vi "ODMR sweep new locked.vi"() -> ()   [LabVIEW 2011]
uses:
  <vilib>/DAQmx/read.llb/DAQmx Read (Counter 1D DBL 1Chan NSamp).vi
  <vilib>/DAQmx/write.llb/DAQmx Write (Digital Bool 1Line 1Point).vi
  <vilib>/DAQmx/create/channels.llb/DAQmx Create Channel (DO-Digital Output).vi
  <vilib>/DAQmx/create/channels.llb/DAQmx Create Channel (CI-Count Edges).vi
  <vilib>/DAQmx/configure/timing.llb/DAQmx Timing (Sample Clock).vi
  <vilib>/Utility/file.llb/Write To Spreadsheet File (DBL).vi
  <vilib>/DAQmx/miscellaneous.llb/DAQmx Fill In Error Info.vi
  Program Files/National Instruments/LabVIEW 2011/resource/objmgr/daqmx.rc
panel:
  out "Frequency":dbl
  in  "Freq max":ext=3300000000.0
  in  "Tracking interval":dbl=150.0
  out "XY Graph":cluster{"Y":dbl[], "Y":dbl[]}[](graph)
  in  "band (1-26.5:2) 2":i32(ring)=2
  in  "resolution (10 Hz:2) 2":i32(ring)=2 items=["0.1 Hz", "1 Hz", "10 Hz", "100 Hz", "1 KHz", "10 KHz", "100 KHz", "1 MHz", "10 MHz", "100 MHz", "1 GHz"]
  in  "GPIB address 2":string="19"
  in  "file path (dialog if empty)":path=path "C:/Users/Ouyang Group/Documents/Calibration pictures/Nanodiamond/1-8-14/X=66 Y=92 Pulse ODMR sweep 4"
  out "Z Position":dbl=31.0
  out "Y Position":dbl=62.0
  out "X Position":dbl=97.0
  in  "Z Pos":dbl=31.0
  in  "Y Pos":dbl=97.0
  in  "X Pos":dbl=62.0
  in  "Y Parameters":T1={"Number of Y Steps"=200, "Max Y (V)"=1.0, "Min Y (V)"=-1.0}
  in  "X Parameters":T2={"Number of X Steps"=200, "Max X (V)"=1.0, "Min X (V)"=-1.0}
  in  "RS232 settings":cluster{"Portnumber":i32, "Baudrate":u16}={"Portnumber"=12, "Baudrate"=5} {"Portnumber" items=["COM1", "COM2", "COM3", "COM4", "COM5", "COM6", "COM7", "COM8", "COM9", "COM10", "COM11", "COM12", "COM13", "COM14", "COM15", "COM16", "COM17", "COM18", "COM19", "COM20", "COM21", "COM22", "COM23", "COM24", "COM25", "COM26", "COM27", "COM28", "COM29", "COM30"]; "Baudrate" items=["9600", "14400", "19200", "38400", "57600", "115200"]}
  in  "samples per channel":i32=500
  in  "rate":dbl=100.0 format="%0.2f"
  in  "stop":bool
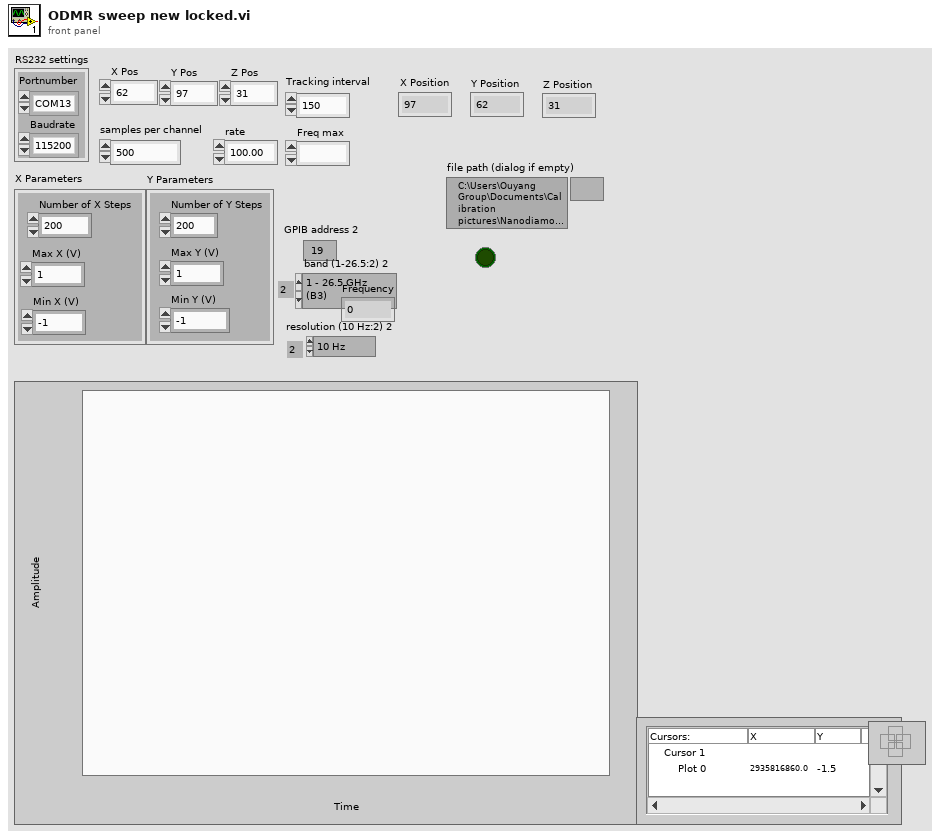
[diagram p1: front panel]
types:
  T1 = cluster{"Number of Y Steps":i32, "Max Y (V)":dbl, "Min Y (V)":dbl}
  T2 = cluster{"Number of X Steps":i32, "Max X (V)":dbl, "Min X (V)":dbl}
  T3 = cluster{"source lock":bool, "lock frequency (Hz)":ext, "coarse tune":bool}
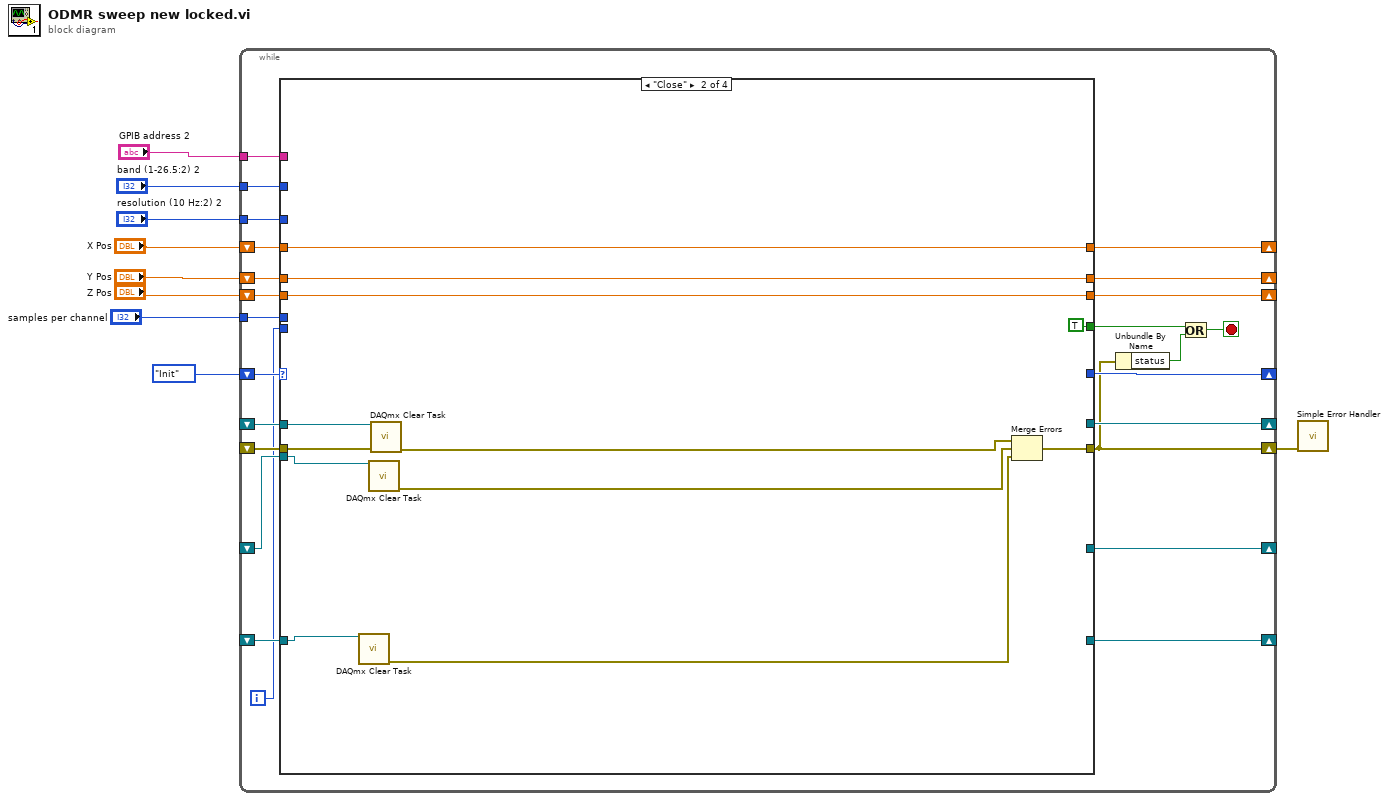
[diagram p0: block diagram]
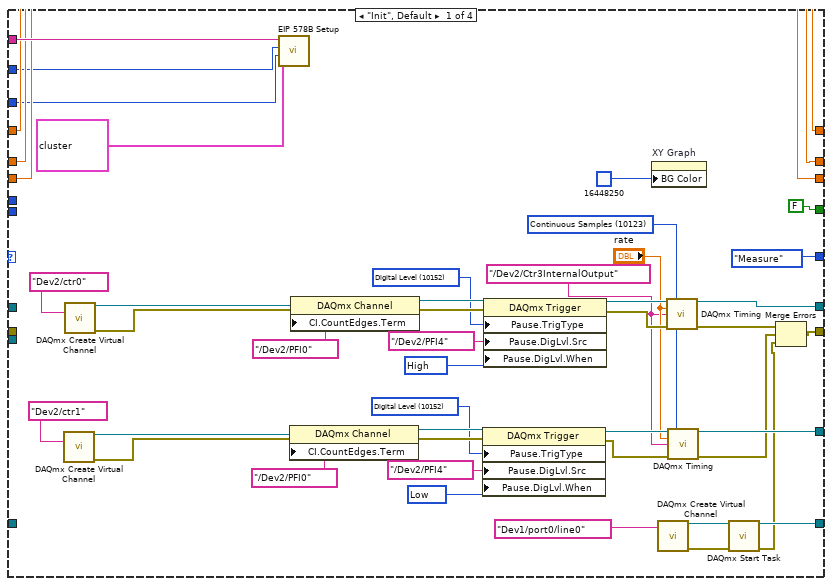
[diagram p2: hidden frame]
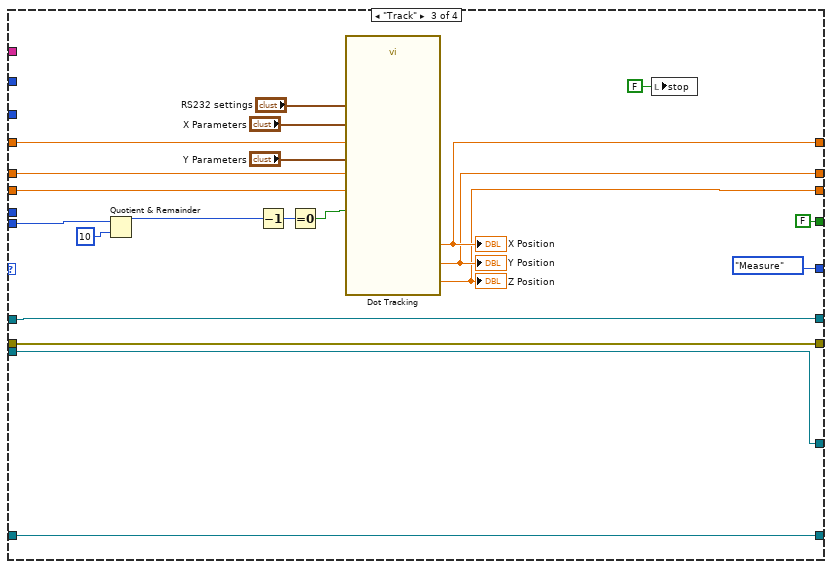
[diagram p3: hidden frame]
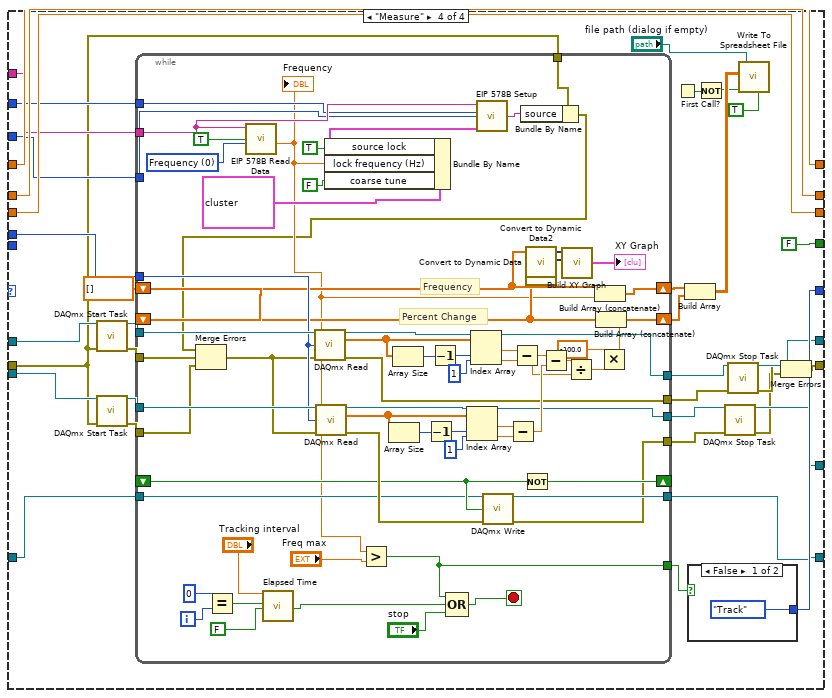
[diagram p4: hidden frame]
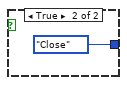
[diagram p5: hidden frame]
diagram:
  n1 = while {
    shift-right: [w29] -> _
    shift-left: enum16{"Init", "Measure", "Track", "Close"}."Init" -> [w33]
    tunnel: "GPIB address 2" -> [w32]
    shift-right: [w31] -> _
    shift-left: _ -> [w28]
    shift-right: [w30] -> _
    shift-left: _ -> [w27]
    shift-right: [w22] -> w6
    shift-left: _ -> [w26]
    shift-right: [w25] -> _
    shift-left: _ -> [w24]
    tunnel: "samples per channel" -> [w19]
    shift-right: [w14] -> _
    shift-left: "X Pos" -> [w17]
    shift-right: [w13] -> _
    shift-left: "Y Pos" -> [w16]
    shift-right: [w12] -> _
    shift-left: "Z Pos" -> [w15]
    tunnel: "band (1-26.5:2) 2" -> [w11]
    tunnel: "resolution (10 Hz:2) 2" -> [w10]
    i -> [w23]
    stop <- w21 stop-if-true
    n2 = case shown="\"Close\"" w33 {
      tunnel: [FALSE TRUE FALSE FALSE] -> w20
      tunnel: w32 -> [w77 _ _ w116]
      tunnel: [w51 _ w111 w134] -> w31
      tunnel: [w50 _ w110 w131] -> w30
      tunnel: [w47 w83 w100 w147] -> w22
      tunnel: [enum16{"Init", "Measure", "Track", "Close"}."Measure" _ enum16{"Init", "Measure", "Track", "Close"}."Measure" w146] -> w29
      tunnel: w28 -> [_ w89 w111 w142]
      tunnel: w27 -> [_ w87 w110 w139]
      tunnel: w26 -> [_ w88 w100 w113]
      tunnel: [w41 _ w109 w135] -> w25
      tunnel: w24 -> [_ w86 w109 w136]
      tunnel: w23 -> [_ _ w101 _]
      tunnel: w19 -> [_ _ _ w121]
      tunnel: w17 -> [w38 w81 w96 w119]
      tunnel: w16 -> [w37 w80 w95 w118]
      tunnel: w15 -> [w36 w79 w94 w117]
      tunnel: [w38 w81 w93 w119] -> w14
      tunnel: [w37 w80 w92 w118] -> w13
      tunnel: [w36 w79 w91 w117] -> w12
      tunnel: w11 -> [w35 _ _ w115]
      tunnel: w10 -> [w34 _ _ w114]
      frame "Init", Default {
        w52 = tag "/Dev2/Ctr3InternalOutput" ("source")
        w54 = 10123 items=["Finite Samples"=10178, "Continuous Samples"=10123, "Hardware Timed Single Point"=12522] ("sample mode")
        w59 = 10214 items=["High"=10192, "Low"=10214] ("Pause.DigLvl.When")
        w61 = 10152 items=["Analog Level"=10101, "Analog Window"=10103, "Digital Level"=10152, "Digital Pattern"=10398, "None"=10230] ("Pause.TrigType")
        w68 = 10192 items=["High"=10192, "Low"=10214] ("Pause.DigLvl.When")
        w70 = 10152 items=["Analog Level"=10101, "Analog Window"=10103, "Digital Level"=10152, "Digital Pattern"=10398, "None"=10230] ("Pause.TrigType")
        n3 = call-poly <vilib>:"DAQmx Create Virtual Channel.vi"("counter"=tag "Dev2/ctr1") -> ("task out"=w66:refnum<k21>, "error out"=w65:errorcluster)  [unwired: 13 in]
        n4 = call-poly <vilib>:"DAQmx Create Virtual Channel.vi"("counter"=tag "Dev2/ctr0") -> ("task out"=w75:refnum<k21>, "error out"=w74:errorcluster)  [unwired: 13 in]
        n5 = call <instrlib>:"EIP 578B Setup.vi"("GPIB Address"=w77, "band (1-26.5 GHz:20)"=w35, "resolution (1 Hz:1)"=w34, "source locking"=T3 {"source lock"=FALSE, "lock frequency (Hz)"=1000000000.0, "coarse tune"=TRUE}) -> ()  [unwired: 2 in, 2 out]
        n6 = property class="DAQmx Channel"(reference=w66, error in=w65, "CI.CountEdges.Term"=tag "/Dev2/PFI0") -> (reference out=w63:refnum<k21>, error out=w62:errorcluster)
        n7 = property class="DAQmx Channel"(reference=w75, error in=w74, "CI.CountEdges.Term"=tag "/Dev2/PFI0") -> (reference out=w72:refnum<k21>, error out=w71:errorcluster)
        n8 = property class="DAQmx Trigger"(reference=w63, error in=w62, "Pause.TrigType"=w61, "Pause.DigLvl.Src"=tag "/Dev2/PFI4", "Pause.DigLvl.When"=w59) -> (reference out=w56:refnum<k21>, error out=w55:errorcluster)
        n9 = property class="DAQmx Trigger"(reference=w72, error in=w71, "Pause.TrigType"=w70, "Pause.DigLvl.Src"=tag "/Dev2/PFI4", "Pause.DigLvl.When"=w68) -> (reference out=w58:refnum<k21>, error out=w57:errorcluster)
        n10 = property on="XY Graph" class="XYGraph (strict)"("BG Color"=u32 16448250) -> ()  [unwired: 2 in, 2 out]
        n11 = call-poly <vilib>:"DAQmx Create Virtual Channel.vi"("lines"=tag "Dev1/port0/line0") -> ("task out"=w43:refnum<k21>, "error out"=w42:errorcluster)  [unwired: 13 in]
        n12 = call-poly <vilib>:"DAQmx Timing.vi"("task/channels in"=w58, "sample mode"=w54, "rate"="rate", "source"=w52, "error in"=w57) -> ("task out"=w51:refnum<k21>, "error out"=w49:errorcluster)  [unwired: 9 in]
        n13 = call-poly <vilib>:"DAQmx Timing.vi"("task/channels in"=w56, "sample mode"=w54, "rate"="rate", "source"=w52, "error in"=w55) -> ("task out"=w50:refnum<k21>, "error out"=w48:errorcluster)  [unwired: 9 in]
        n14 = call <vilib>:"DAQmx Start Task.vi"("task/channels in"=w43, "error in"=w42) -> ("task out"=w41:refnum<k21>, "error out"=w40:errorcluster)  [unwired: 12 in]
        n15 = Merge Errors(w49, w48, w40) -> (w47:errorcluster)
      }
      frame "Close" {
        n16 = call <vilib>:"DAQmx Clear Task.vi"("task in"=w86) -> ("error out"=w84:errorcluster)  [unwired: 14 in]
        n17 = call <vilib>:"DAQmx Clear Task.vi"("task in"=w87) -> ("error out"=w85:errorcluster)  [unwired: 14 in]
        n18 = call <vilib>:"DAQmx Clear Task.vi"("task in"=w89, "error in"=w88) -> ("error out"=w82:errorcluster)  [unwired: 13 in]
        n19 = Merge Errors(w82, w85, w84) -> (w83:errorcluster)
      }
      frame "Track" {
        n20 = Quotient & Remainder(x=w101, y=10) -> (x-y*floor(x/y)=w104:i32)  [unwired: 1 out]
        n21 = Decrement(x=w104) -> (x-1=w105:i32)
        n22 = Equal To 0?(x=w105) -> (x = 0?=w102:bool)
        n23 = call "Dot Tracking.vi"("X Parameters"="X Parameters", "Y Parameters"="Y Parameters", "RS232 settings"="RS232 settings", "X Pos"=w96, "Y pos"=w95, "Z Pos"=w94, "Z-track?"=w102) -> ("X Position"=w93:dbl, "Y Position"=w92:dbl, "Z Position"=w91:dbl)  [unwired: 2 in, 4 out]
        "X Position" <- w93
        "Y Position" <- w92
        "Z Position" <- w91
        n24 = local write "stop"(FALSE ("stop")) -> ()
      }
      frame "Measure" {
        w120 = dbl[] []
        n25 = call <vilib>:"DAQmx Start Task.vi"("task/channels in"=w142, "error in"=w113) -> ("task out"=w140:refnum<k21>, "error out"=w141:errorcluster)  [unwired: 12 in]
        n26 = call <vilib>:"DAQmx Start Task.vi"("task/channels in"=w139, "error in"=w113) -> ("task out"=w138:refnum<k21>, "error out"=w137:errorcluster)  [unwired: 12 in]
        n27 = while {
          shift-right: [w199] -> w127
          shift-left: w120 -> [w179]
          shift-right: [w198] -> w128
          shift-left: w120 -> [w181]
          shift-right: [w192] -> _
          shift-left: _ -> [w193]
          tunnel: w138 -> [w191]
          tunnel: [w190] -> w133
          tunnel: [w189] -> w144
          tunnel: [w184] -> w143
          tunnel: w141 -> [w188]
          tunnel: w140 -> [w187]
          tunnel: w137 -> [w152]
          tunnel: w136 -> [w186]
          tunnel: [w185] -> w135
          tunnel: [w183] -> w130
          tunnel: w121 -> [w182]
          tunnel: w116 -> [w166]
          tunnel: w115 -> [w165]
          tunnel: w114 -> [w164]
          tunnel: w113 -> [w155]
          tunnel: [w150] -> w112
          i -> [w168]
          stop <- w156 stop-if-true
          w172 = 0 items=["Frequency", "Power", "Both"] ("output mode (freq:0)")
          # "Percent Change"
          # "Frequency"
          n28 = Equal?(x=0, y=w168) -> (x = y?=w167:bool)
          n29 = call <instrlib>:"EIP 578B Read Data.vi"("output mode (freq:0)"=w172, "fast (T=active)"=TRUE, "GPIB"=w166) -> ("frequency (Hz)"=w159:ext)  [unwired: 1 in, 3 out]
          "Frequency" <- w159
          n30 = call "Elapsed Time"("Time Target (s)"="Tracking interval", "Reset"=w167, "Auto Reset"=FALSE) -> ("Time has Elapsed"=w158:bool)  [unwired: 9 in, 7 out]
          n31 = Bundle By Name(cluster=T3 {"source lock"=FALSE, "lock frequency (Hz)"=1000000000.0, "coarse tune"=TRUE} ("source locking"), "source lock"=TRUE, "lock frequency (Hz)"=w159, "coarse tune"=FALSE) -> (w160:T3)
          n32 = Greater?(x=w159, y="Freq max") -> (0:w150:bool)
          n33 = Compound Arithmetic op=OR(w150, w158, "stop") -> (w156:bool)
          n34 = call <instrlib>:"EIP 578B Setup.vi"("GPIB Address"=w166, "band (1-26.5 GHz:20)"=w165, "resolution (1 Hz:1)"=w164, "source locking"=w160) -> ("status messages"=w154:string)  [unwired: 2 in, 1 out]
          n35 = Bundle By Name(cluster=w155, "source"=w154) -> (w153:errorcluster)
          n36 = Merge Errors(w153, w188, w152) -> (w151:errorcluster)
          n37 = call-poly <vilib>:"DAQmx Read.vi"("task/channels in"=w187, "number of samples per channel"=w182, "error in"=w151) -> ("task out"=w189:refnum<k21>, "data"=w212:dbl[], "error out"=w190:errorcluster)  [unwired: 10 in]
          n38 = call-poly <vilib>:"DAQmx Read.vi"("task/channels in"=w191, "number of samples per channel"=w182, "error in"=w151) -> ("task out"=w184:refnum<k21>, "data"=w201:dbl[], "error out"=w194:errorcluster)  [unwired: 10 in]
          n39 = Array Size(array=w201) -> (size(s)=w206:i32)
          n40 = Array Size(array=w212) -> (size(s)=w211:i32)
          n41 = Decrement(x=w206) -> (x-1=w205:i32)
          n42 = Decrement(x=w211) -> (x-1=w210:i32)
          n43 = Index Array(array=w201, index #1=w205, index #2=1 ("index")) -> (element #1=w202:dbl, element #2=w203:dbl)
          n44 = Index Array(array=w212, index #1=w210, index #2=1 ("index")) -> (element #1=w207:dbl, element #2=w208:dbl)
          n45 = call-poly <vilib>:"DAQmx Write.vi"("task/channels in"=w186, "data"=w193, "error in"=w194) -> ("task out"=w185:refnum<k21>, "error out"=w183:errorcluster)  [unwired: 10 in, 1 out]
          n46 = Subtract(x=w202, y=w203) -> (x-y=w200:dbl)
          n47 = Subtract(x=w207, y=w208) -> (x-y=w196:dbl)
          n48 = Not(x=w193) -> (.not. x?=w192:bool)
          n49 = call "Convert to Dynamic Data"("Array"=w181) -> ("Dynamic Data Type"=w180:dynamicdata)  [unwired: 3 in]
          n50 = call "Convert to Dynamic Data2"("Array"=w179) -> ("Dynamic Data Type"=w178:dynamicdata)  [unwired: 3 in]
          n51 = Subtract(x=w196, y=w200) -> (x-y=w197:dbl)
          n52 = call "Build XY Graph"("Y Input"=w178, "X Input"=w180) -> ("XY Graph"=→"XY Graph":cluster{"Y":dbl[], "Y":dbl[]}[])  [unwired: 3 in, 6 out]
          n53 = Divide(x=w197, y=w196) -> (x/y=w195:dbl)
          n54 = Build Array (concatenate)(w181, w159) -> (w198:ext[])
          n55 = Multiply(x=-100.0, y=w195) -> (x*y=w176:dbl)
          n56 = Build Array (concatenate)(w179, w176) -> (w199:dbl[])
        }
        n57 = First Call?() -> (First Call?: T/F=w125:bool)
        n58 = Build Array(w128, w127) -> (w126:ext[][])
        n59 = case shown="False" w112 {
          tunnel: [enum16{"Init", "Measure", "Track", "Close"}."Track" enum16{"Init", "Measure", "Track", "Close"}."Close"] -> w146
          frame False {
          }
          frame True {
          }
        }
        n60 = Not(x=w125) -> (.not. x?=w124:bool)
        n61 = call <vilib>:"DAQmx Stop Task.vi"("task/channels in"=w143, "error in"=w130) -> ("task out"=w131:refnum<k21>, "error out"=w129:errorcluster)  [unwired: 12 in]
        n62 = call <vilib>:"DAQmx Stop Task.vi"("task/channels in"=w144, "error in"=w133) -> ("task out"=w134:refnum<k21>, "error out"=w132:errorcluster)  [unwired: 12 in]
        n63 = call-poly <vilib>:"Write To Spreadsheet File.vi"("transpose? (no:F)"=TRUE, "append to file? (new file:F)"=w124, "2D data"=w126, "file path (dialog if empty)"="file path (dialog if empty)") -> ()  [unwired: 4 in, 1 out]
        n64 = Merge Errors(w132, w129) -> (w147:errorcluster)
      }
    }
    n65 = Unbundle By Name(w22) -> ("status"=w18:bool)
    n66 = Or(x=w20, y=w18) -> (x .or. y?=w21:bool)
  }
  n67 = call <vilib>:"Simple Error Handler.vi"("error in (no error)"=w6) -> ()  [unwired: 4 in, 5 out]
